vi "Indentation level.vi"(0 "String":string) -> (1 "Spaces Before Key":string, 2 "length":i32, 3 "Level":u32)   [LabVIEW 2015, in "YAML Parser.lvclass"]
uses:
  YAML Parser.lvclass
  <vilib>/regexp/Match Regular Expression.xnode
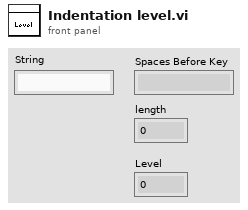
[diagram p1: front panel]
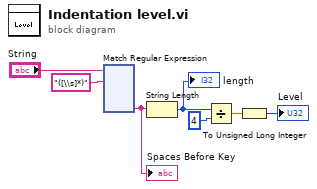
[diagram p0: block diagram]
diagram:
  n1 = xnode "Match Regular Expression"("input string"="String", "regular expression"="([\\s]*)") -> ("submatch 1"=w4:string)  [unwired: 4 in, 5 out]
  "Spaces Before Key" <- w4
  n2 = String Length(string=w4) -> (length=w3:i32)
  "length" <- w3
  n3 = Divide(x=w3, y=4) -> (x/y=w5:dbl)
  n4 = To Unsigned Long Integer(number=w5) -> (unsigned 32bit integer=→"Level":u32)
